vi "MovemotorMeng2.vi"(8 "error in (no error)":errorcluster, 9 "change":i32, 10 "direction":u32, 11 "Automation Refnum in":refnum<k7>) -> (0 "error out":errorcluster, 1 "Position":sgl, 3 "Automation Refnum out":refnum<k7>)   [LabVIEW 2014]
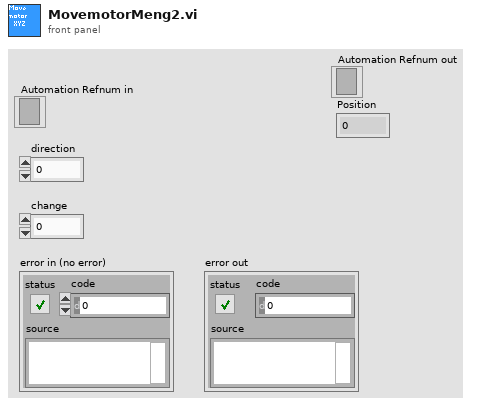
[diagram p1: front panel]
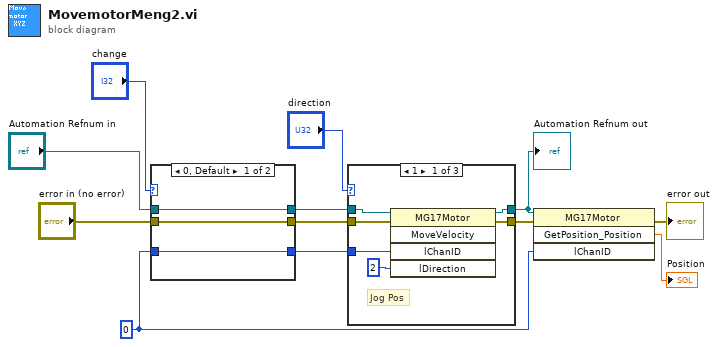
[diagram p0: block diagram]
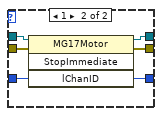
[diagram p2: hidden frame]
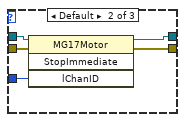
[diagram p3: hidden frame]
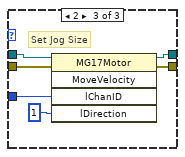
[diagram p4: hidden frame]
diagram:
  w2 = 0 ("lChanID")
  n1 = case shown="0, Default" "change" {
    tunnel: "Automation Refnum in" -> [w15 w21]
    tunnel: [w15 w20] -> w5
    tunnel: "error in (no error)" -> [w14 w19]
    tunnel: [w14 w18] -> w3
    tunnel: w2 -> [w13 w17]
    tunnel: [w13 w16] -> w1
    frame 0, Default {
    }
    frame 1 {
      n2 = invoke class="MG17Motor" method="StopImmediate"(reference=w21, error in=w19, "lChanID"=w17) -> (reference out=w20:refnum<k7>, error out=w18:errorcluster, "lChanID"=w16:i32)  [unwired: 1 in, 1 out]
    }
  }
  n3 = case shown="1" "direction" {
    tunnel: [w27 w32 w38] -> w11
    tunnel: [w25 w31 w36] -> w10
    tunnel: w5 -> [w24 w30 w35]
    tunnel: w3 -> [w23 w29 w34]
    tunnel: w1 -> [w22 w28 w33]
    frame 1 {
      # "Jog Pos"
      n4 = invoke class="MG17Motor" method="MoveVelocity"(reference=w24, error in=w23, "lChanID"=w22, "lDirection"=2) -> (reference out=w25:refnum<k7>, error out=w27:errorcluster)  [unwired: 1 in, 3 out]
    }
    frame Default {
      n5 = invoke class="MG17Motor" method="StopImmediate"(reference=w30, error in=w29, "lChanID"=w28) -> (reference out=w31:refnum<k7>, error out=w32:errorcluster)  [unwired: 1 in, 2 out]
    }
    frame 2 {
      # "Set Jog Size"
      n6 = invoke class="MG17Motor" method="MoveVelocity"(reference=w35, error in=w34, "lChanID"=w33, "lDirection"=1) -> (reference out=w36:refnum<k7>, error out=w38:errorcluster)  [unwired: 1 in, 3 out]
    }
  }
  "Automation Refnum out" <- w10
  n7 = invoke class="MG17Motor" method="GetPosition_Position"(reference=w10, error in=w11, "lChanID"=w2) -> (error out=→"error out":errorcluster, "GetPosition_Position"=→"Position":sgl)  [unwired: 1 in, 2 out]
